vi "Reactive_philosopher.vi"(5 "Maximum attempts":i32, 6 "Maximum think time":u32=1000, 7 "Maximum eat time":u32=1000, 9 "total":i32, 10 "Ph id":i32) -> ()   [LabVIEW 2015]
uses:
  SINGLE_CHOP_Separator_string.ctl
  CHOPS_COUPLE_separator_string.ctl
panel:
  out "concatenated string":string
  # "Viene LANCIATO DA PHILOSOFERS"
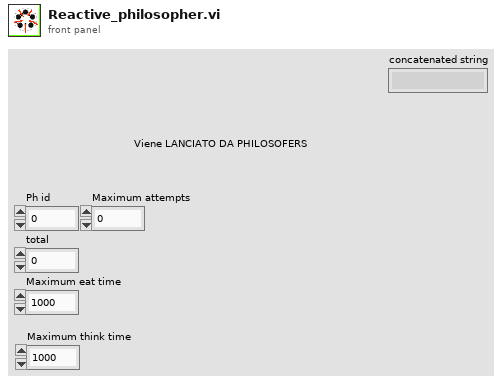
[diagram p1: front panel]
types:
  T1 = typedef "CHOPS_COUPLE_separator_string.ctl" = string
  T2 = typedef "SINGLE_CHOP_Separator_string.ctl" = string
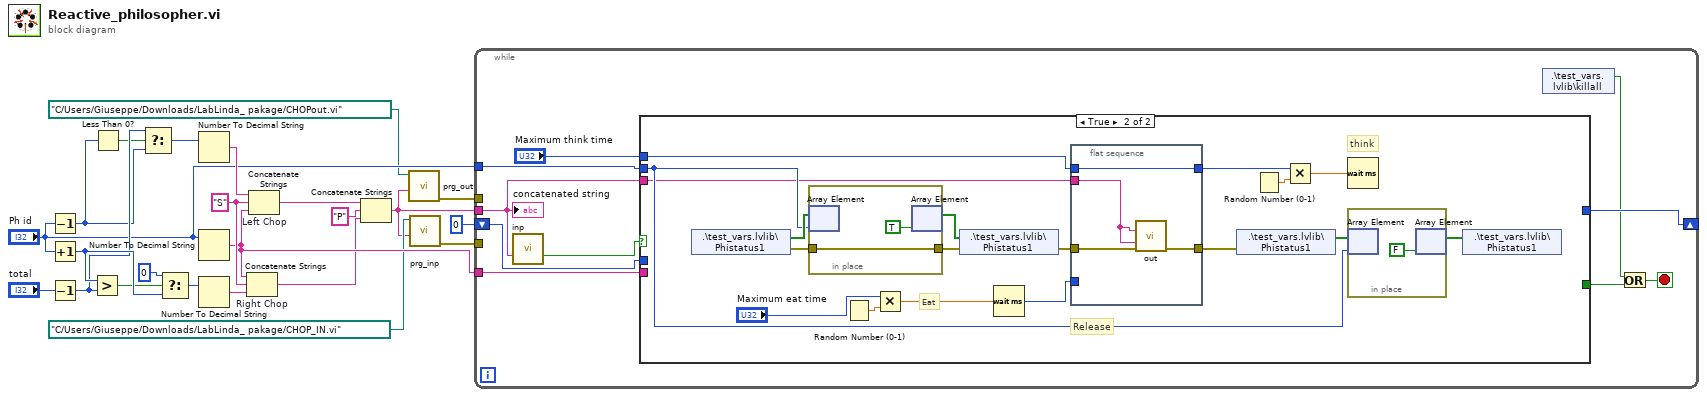
[diagram p0: block diagram]
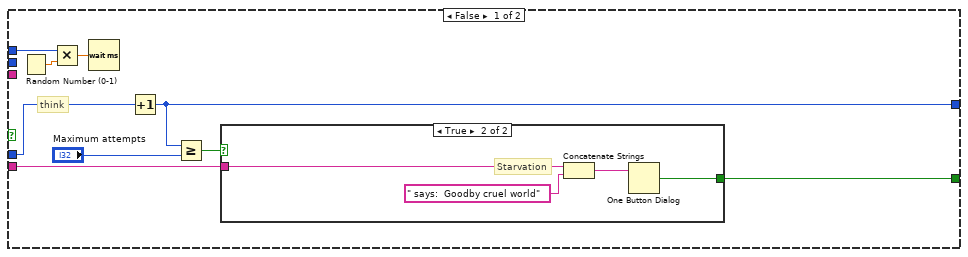
[diagram p2: hidden frame]
diagram:
  w15 = T2 "S"
  n1 = Decrement(x="Ph id") -> (x-1=w13:i32)
  n2 = Increment(x="Ph id") -> (x+1=w20:i32)
  n3 = Decrement(x="total") -> (x-1=w18:i32)
  n4 = Greater?(x=w20, y=w18) -> (0:w19:bool)
  n5 = Less Than 0?(x=w13) -> (x < 0?=w12:bool)
  n6 = Select(t=w18, s=w12, f=w13) -> (s? t:f=w14:i32)
  n7 = Select(t=0, s=w19, f=w20) -> (s? t:f=w22:i32)
  n8 = Number To Decimal String(number=w14) -> (decimal integer string=w17:string)  [unwired: 1 in]
  n9 = Number To Decimal String(number="Ph id") -> (decimal integer string=w9:string)  [unwired: 1 in]
  n10 = Number To Decimal String(number=w22) -> (decimal integer string=w16:string)  [unwired: 1 in]
  n11 = Concatenate Strings "Right Chop"(w9, w15, w16) -> (w6:string)
  n12 = Concatenate Strings "Left Chop"(w17, w15, w9) -> (w7:string)
  n13 = Concatenate Strings(w7, T1 "P" ("search string/char (-)"), w6) -> (w3:string)
  n14 = call "prg_out.vi"("Name"=w3, "vi path"=path "C:/Users/Giuseppe/Downloads/LabLinda_ pakage/CHOPout.vi") -> ("error out"=w1:errorcluster)  [unwired: 9 in]
  n15 = call "prg_inp.vi"("Name"=w3, "vi path"=path "C:/Users/Giuseppe/Downloads/LabLinda_ pakage/CHOP_IN.vi") -> ("error out"=w4:errorcluster)  [unwired: 9 in]
  n16 = while {
    shift-right: [w32] -> _
    shift-left: 0 -> [w33]
    tunnel: "Ph id" -> [w27]
    tunnel: w9 -> [w26]
    tunnel: w4 -> [_]
    tunnel: w3 -> [w25]
    tunnel: w1 -> [_]
    stop <- w29 stop-if-true
    n17 = call "inp.vi"("Name in"=w25) -> ("Valid data"=w24:bool)  [unwired: 12 in, 2 out]
    n18 = case shown="True" w24 {
      tunnel: w33 -> [w42 _]
      tunnel: [w39 _] -> w28
      tunnel: [w38 _] -> w32
      tunnel: w26 -> [w35 _]
      tunnel: "Maximum think time" -> [w34 w50]
      tunnel: w27 -> [_ w55]
      tunnel: w25 -> [_ w48]
      frame False {
        # "think"
        n19 = Random Number (0-1)() -> (number: 0 to 1=w37:dbl)
        n20 = Multiply(x=w34, y=w37) -> (x*y=w36:dbl)
        n21 = Wait (ms)(milliseconds to wait=w36) -> ()  [unwired: 1 out]
        n22 = Increment(x=w42) -> (x+1=w38:i32)
        n23 = Greater Or Equal?(x=w38, y="Maximum attempts") -> (x >= y?=w40:bool)
        n24 = case shown="True" w40 {
          tunnel: [_ w46] -> w39
          tunnel: w35 -> [_ w45]
          frame False {
          }
          frame True {
            # "Starvation"
            n25 = Concatenate Strings(w45, " says:  Goodby cruel world" ("message")) -> (w43:string)
            n26 = One Button Dialog(message=w43) -> (true=w46:bool)  [unwired: 1 in]
          }
        }
      }
      frame True {
        # "Release"
        # "think"
        # "Eat"
        n27 = shared-variable ".\\test_vars.lvlib\\Phistatus1"() -> (w59:bool[], error out=w54:errorcluster)  [unwired: 1 in]
        n28 = in-place {
          in-place-border: w54 -> [w70]
          in-place-border: [w70] -> w53
          n29 = in-place-array #1(w59, w55) -> ()  [unwired: 1 out]
          n30 = in-place-array #1(TRUE ("element")) -> (w58:bool[])  [unwired: 1 out]
        }
        n31 = Random Number (0-1)() -> (number: 0 to 1=w64:dbl)
        n32 = Multiply(x="Maximum eat time", y=w64) -> (x*y=w62:dbl)
        n33 = shared-variable ".\\test_vars.lvlib\\Phistatus1"(w58, error in=w53) -> (error out=w52:errorcluster)
        n34 = Wait (ms)(milliseconds to wait=w62) -> (millisecond timer value=w47:u32)
        n35 = flat-sequence {
          tunnel: w52 -> [w67]
          tunnel: [w66] -> w51
          tunnel: w48 -> [w65]
          tunnel: w50 -> [w68]
          tunnel: [w68] -> w49
          tunnel: w47 -> [_]
          frame #0 {
            n36 = call "out.vi"("IN VARIANT"=w65, "Name in"=w65, "error in (no error)"=w67) -> ("error out"=w66:errorcluster)  [unwired: 11 in, 1 out]
          }
        }
        n37 = shared-variable ".\\test_vars.lvlib\\Phistatus1"(error in=w51) -> (w56:bool[])  [unwired: 1 out]
        n38 = Random Number (0-1)() -> (number: 0 to 1=w61:dbl)
        n39 = Multiply(x=w49, y=w61) -> (x*y=w60:dbl)
        n40 = Wait (ms)(milliseconds to wait=w60) -> ()  [unwired: 1 out]
        n41 = in-place {
          n42 = in-place-array #2(w56, w55) -> ()  [unwired: 1 out]
          n43 = in-place-array #2(FALSE ("element")) -> (w57:bool[])  [unwired: 1 out]
        }
        n44 = shared-variable ".\\test_vars.lvlib\\Phistatus1"(w57) -> ()  [unwired: 1 in, 1 out]
      }
    }
    n45 = shared-variable ".\\test_vars.lvlib\\killall"() -> (w30:bool)  [unwired: 1 in, 1 out]
    n46 = Or(x=w30, y=w28) -> (x .or. y?=w29:bool)
    "concatenated string" <- w25
  }
